vi "Configure Event Search (Transition).vi"(6 "Transition Time (2E-8 S)":dbl=2e-08, 7 "Edge Slope (0: Positive)":i32(ring) items=["Positive", "Negative"], 8 "error in (no error)":errorcluster, 9 "Qualifier (1: Less)":i32(ring)=1 items=["Greater", "Less"], 10 "Source Channel (0: Channel 1)":i32(ring) items=["Channel 1", "Channel 2", "Channel 3", "Channel 4"], 11 "VISA resource name":refnum<visa-resource-name>) -> (0 "error out":errorcluster, 3 "VISA resource name out":refnum<visa-resource-name>)   [LabVIEW 2015, in "Agilent 2000 3000 X-Series.lvlib"]
doc: "Configures the event search of Transition."
uses:
  <instrlib>/Agilent 2000 3000 X-Series/Agilent 2000 3000 X-Series.lvlib
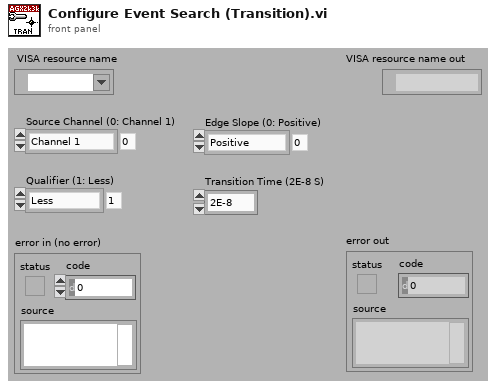
[diagram p1: front panel]
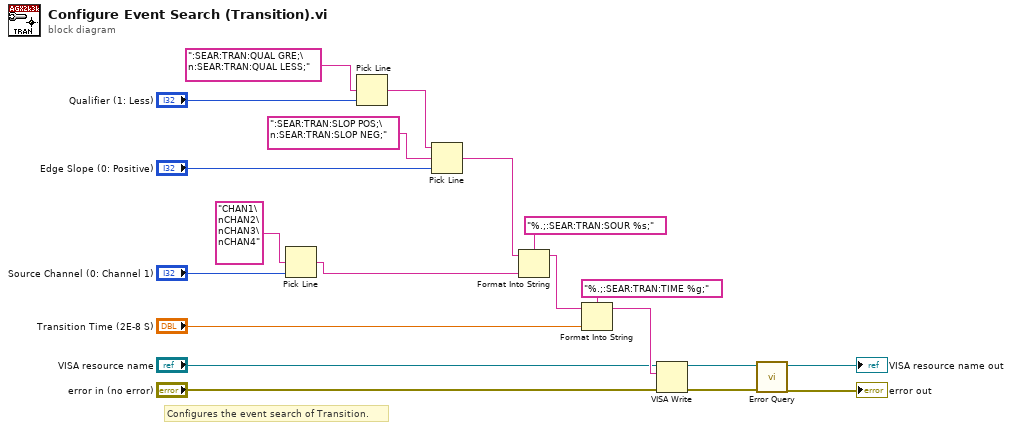
[diagram p0: block diagram]
diagram:
  # "Configures the event search of Transition."
  n1 = Pick Line(multi-line string="CHAN1\nCHAN2\nCHAN3\nCHAN4", line index="Source Channel (0: Channel 1)") -> (output string=w1:string)  [unwired: 1 out]
  n2 = Pick Line(multi-line string=":SEAR:TRAN:QUAL GRE;\n:SEAR:TRAN:QUAL LESS;", line index="Qualifier (1: Less)") -> (output string=w16:string)  [unwired: 1 out]
  n3 = Pick Line(string ("")=w16, multi-line string=":SEAR:TRAN:SLOP POS;\n:SEAR:TRAN:SLOP NEG;", line index="Edge Slope (0: Positive)") -> (output string=w6:string)
  n4 = Format Into String(format string="%.;:SEAR:TRAN:SOUR %s;", initial string=w6, w1) -> (resulting string=w4:string)  [unwired: 1 in, 1 out]
  n5 = Format Into String(format string="%.;:SEAR:TRAN:TIME %g;", initial string=w4, "Transition Time (2E-8 S)") -> (resulting string=w13:string)  [unwired: 1 in, 1 out]
  n6 = VISA Write(VISA resource name="VISA resource name", write buffer=w13, error in (no error)="error in (no error)") -> (VISA resource name out=w10:refnum<visa-resource-name>, error out=w9:errorcluster)  [unwired: 1 out]
  n7 = call <instrlib>:"Error Query.vi"("error in (no error)"=w9, "VISA resource name"=w10) -> ("error out"=→"error out":errorcluster, "VISA resource name out"=→"VISA resource name out":refnum<visa-resource-name>)  [unwired: 8 out]
